vi "HelperVI-keyboardsimulation.vi"() -> ()   [LabVIEW 2016, in "DronaTest.lvlib" / "test_ValueSignal.lvlib"]
uses:
  test_ValueSignal.lvlib
panel:
  in  "Stop":bool
  in  "Boolean":bool
  in  "Tab Control":enum32{"Page 1", "Page 2"}(tab)
  in  "String":string
  in  "Numeric":dbl
  in  "Cluster":T1
  in  "String":string
  in  "Numeric":dbl
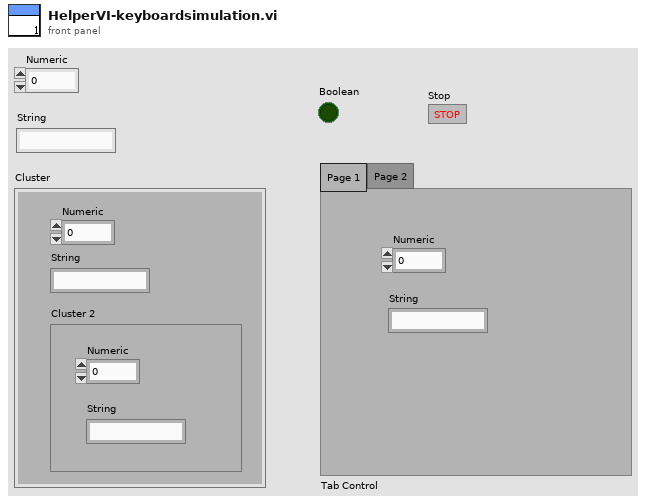
[diagram p1: front panel]
types:
  T1 = cluster{"Numeric":dbl, "String":string, "Cluster 2":cluster{"Numeric":dbl, "String":string}}
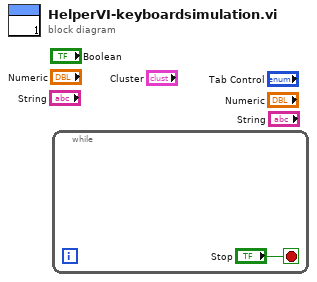
[diagram p0: block diagram]
diagram:
  n1 = while {
    stop <- "Stop" stop-if-true
  }
